vi "PARAM_REQUEST_READ.vi"(10 "Target System and Target Component":u8=1, 11 "param_id":string) -> (3 "MAVLink Message":u8[](array[numeric]))   [LabVIEW 2014]
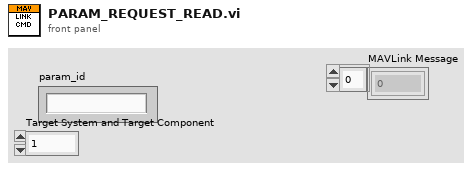
[diagram p1: front panel]
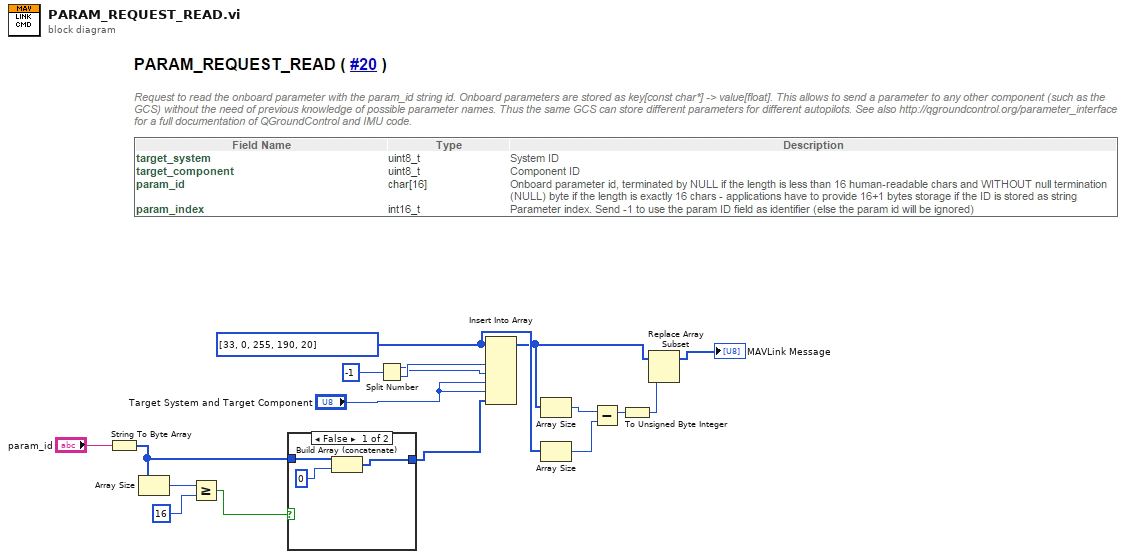
[diagram p0: block diagram]
diagram:
  w16 = u8[] [33, 0, 255, 190, 20]
  n1 = String To Byte Array(string="param_id") -> (unsigned byte array=w3:u8[])
  n2 = Array Size(array=w3) -> (size(s)=w6:i32)
  n3 = Greater Or Equal?(x=w6, y=16) -> (x >= y?=w4:bool)
  n4 = case shown="False" w4 {
    tunnel: [w18 w21] -> w2
    tunnel: w3 -> [w20 w21]
    frame False {
      n5 = Build Array (concatenate)(w20, u8 0) -> (w18:u8[])
    }
    frame True {
    }
  }
  n6 = Split Number(x=i16 -1) -> (hi(x)=w8:u8, lo(x)=w9:u8)
  n7 = Insert Into Array(array=w16, new element #1=w9, new element #2=w8, new element #3="Target System and Target Component", new element #4="Target System and Target Component", new element #5=w2) -> (w14:u8[])  [unwired: 1 in]
  n8 = Array Size(array=w14) -> (size(s)=w17:i32)
  n9 = Array Size(array=w16) -> (size(s)=w15:i32)
  n10 = Subtract(x=w17, y=w15) -> (x-y=w12:i32)
  n11 = To Unsigned Byte Integer(number=w12) -> (unsigned 8bit integer=w11:u8)
  n12 = Replace Array Subset(array=w14, new element=w11) -> (→"MAVLink Message":u8[])  [unwired: 1 in]
